vi "medicion.vi"(8 "Powermeter":T1={"Readout Config"="POW", "tiempo. lect."=0.0, "num. med"=0.0}, 9 "Config. fotodiodo":cluster{"tiempo. lect.":dbl, "num. med":dbl}, 10 "config. Polarizador":T2, 11 "Config. voltaje y corriente":T3 {"Measurement Function (0:Voltage)" items=["Voltage", "Current", "Power"]; "Unit(V)" items=["V", "mV", "kV", "A", "mA"]; "Function(0:Voltage)" items=["Voltage", "Current"]}) -> (0 "LockIn":dbl, 1 "Valor voltaje":dbl, 2 "Power meter":cluster{dbl[], dbl[]}(graph), 3 "Fototubo":cluster{dbl[], dbl[]}(graph), 4 "Readout value":dbl format="%^#_9e")   [LabVIEW 2016]
uses:
  <vilib>/Analysis/baseanly.llb/Mean (DBL).vi
  <instrlib>/Keithley 2200 Series/Keithley 2200 Series.lvlib
  <vilib>/Analysis/NI_AALBase.lvlib
panel:
  out "Readout string":string
  out "New":bool
  out "Error log":string
  in  "stop":bool
  out "name":string
  out "flags":bool[](array[boolean])
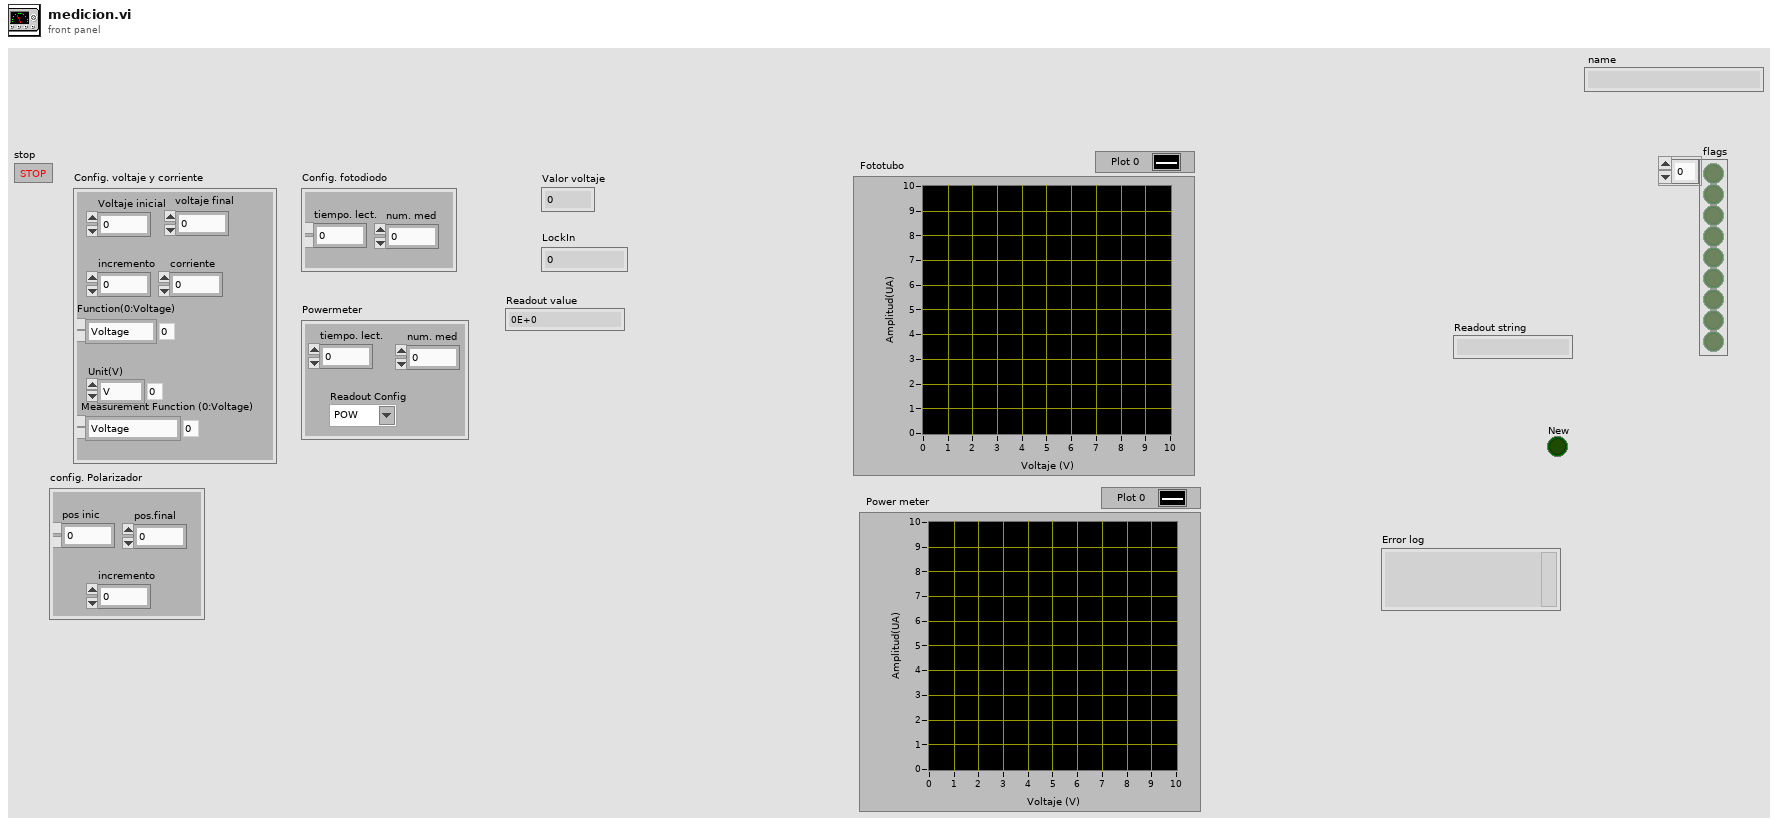
[diagram p1: front panel]
types:
  T1 = cluster{"Readout Config":string, "tiempo. lect.":dbl, "num. med":dbl}
  T2 = cluster{"pos inic":dbl, "pos.final":dbl, "incremento":dbl}
  T3 = cluster{"Voltaje inicial":dbl, "incremento":dbl, " voltaje final":dbl, "corriente":dbl, "Function(0:Voltage)":u16, "Unit(V)":u16, "Measurement Function (0:Voltage)":u16}
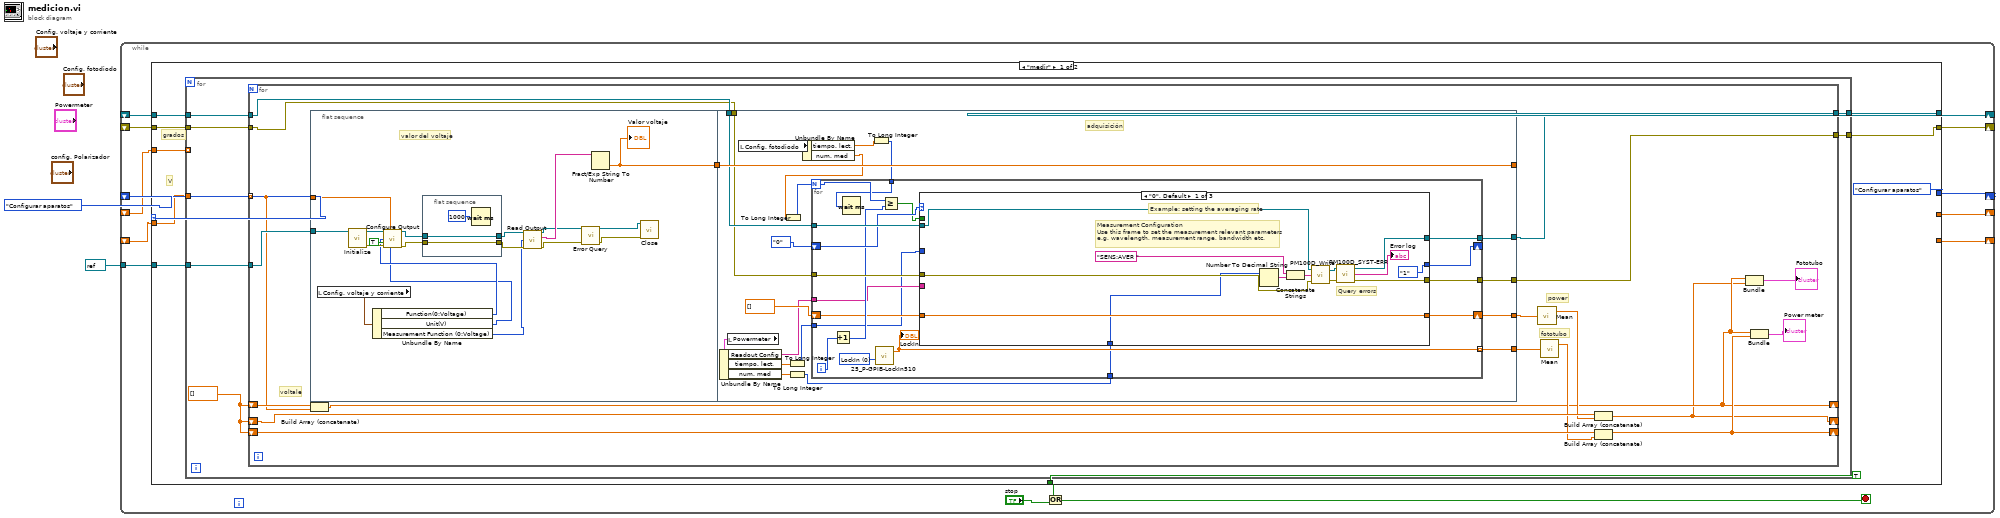
[diagram p0: block diagram]
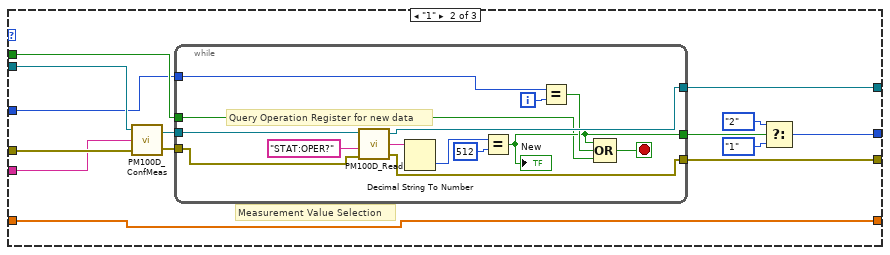
[diagram p2: hidden frame]
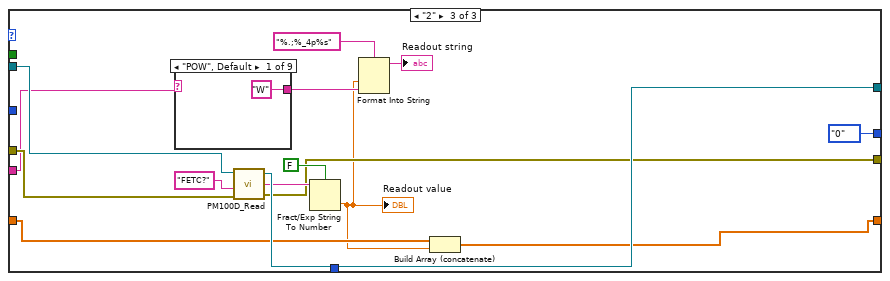
[diagram p3: hidden frame]
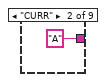
[diagram p4: hidden frame]
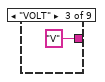
[diagram p5: hidden frame]
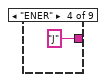
[diagram p6: hidden frame]
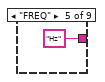
[diagram p7: hidden frame]
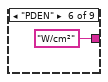
[diagram p8: hidden frame]
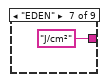
[diagram p9: hidden frame]
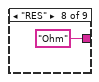
[diagram p10: hidden frame]
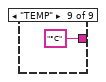
[diagram p11: hidden frame]
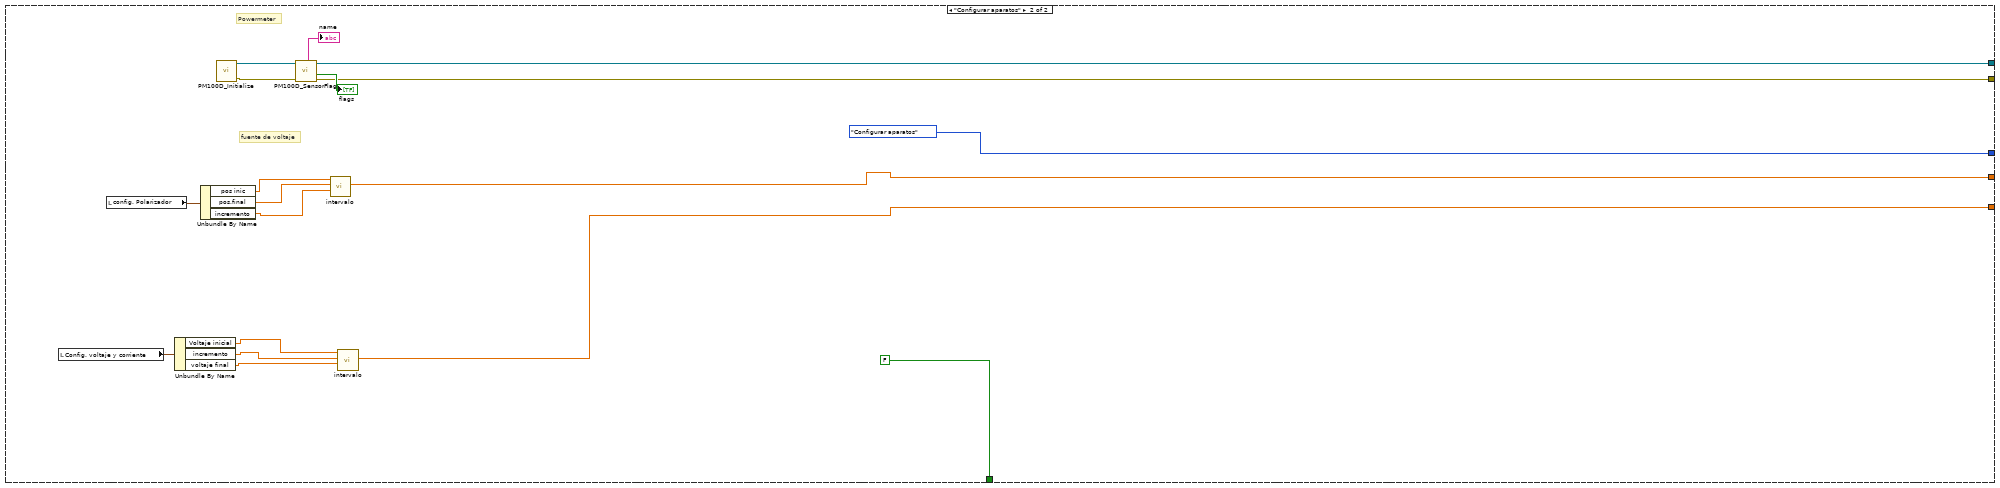
[diagram p12: hidden frame]
diagram:
  n1 = while {
    shift-right: [w3] -> _
    shift-left: enum16{"Configurar aparatos", "medir"}."Configurar aparatos" -> [w16]
    shift-right: [w15] -> _
    shift-left: _ -> [w9]
    shift-right: [w14] -> _
    shift-left: _ -> [w8]
    shift-right: [w13] -> _
    shift-left: _ -> [w11]
    shift-right: [w12] -> _
    shift-left: _ -> [w10]
    tunnel: refnum<visa-resource-name> refnum ("VISA resource name") -> [w4]
    stop <- w7 stop-if-true
    n2 = case shown="\"medir\"" w16 {
      tunnel: [w18 w184] -> w15
      tunnel: [w17 w183] -> w14
      tunnel: [_ w182] -> w13
      tunnel: [_ w181] -> w12
      tunnel: w11 -> [w25 _]
      tunnel: w10 -> [w24 _]
      tunnel: w9 -> [w23 _]
      tunnel: w8 -> [w22 _]
      tunnel: [TRUE FALSE] -> w5
      tunnel: w4 -> [w20 _]
      tunnel: [enum16{"Configurar aparatos", "medir"}."Configurar aparatos" enum16{"Configurar aparatos", "medir"}."Configurar aparatos"] -> w3
      frame "medir" {
        # "V"
        # "grados"
        n3 = for {
          tunnel: w25 -> [_] mode=indexing
          tunnel: w24 -> [w32]
          tunnel: w23 -> [w31]
          tunnel: w22 -> [w30]
          tunnel: w20 -> [w29]
          tunnel: [w27] -> w18
          tunnel: [w26] -> w17
          w28 = dbl[] []
          n4 = for {
            tunnel: w32 -> [w49] mode=indexing
            tunnel: w31 -> [w47]
            tunnel: w30 -> [w46]
            tunnel: w29 -> [w51]
            shift-right: [w34] -> _
            shift-left: w28 -> [w50]
            shift-right: [w33] -> _
            shift-left: w28 -> [w43]
            shift-right: [w36] -> _
            shift-left: w28 -> [w42]
            tunnel: [w39] -> w27
            tunnel: [w38] -> w26
            # "fototubo"
            # "power"
            # "voltale"
            n5 = flat-sequence {
              tunnel: w49 -> [w61]
              tunnel: w51 -> [w70]
              tunnel: [w60] -> w48
              tunnel: w48 -> [w93]
              tunnel: w47 -> [w89]
              tunnel: w46 -> [w88]
              tunnel: [w93] -> _
              tunnel: [w77] -> w45
              tunnel: [w76] -> w44
              tunnel: [w75] -> w39
              tunnel: [w74] -> w38
              frame #0 {
                # "valor del voltaje"
                n6 = local read "Config. voltaje y corriente"() -> (w59:T3)
                n7 = call <instrlib>:"Initialize.vi"("VISA resource name"=w70) -> ("error out"=w68:errorcluster, "VISA resource name out"=w69:refnum<visa-resource-name>)  [unwired: 9 in]
                n8 = Unbundle By Name(w59) -> ("Function(0:Voltage)"=w58:u16, "Unit(V)"=w57:u16, "Measurement Function (0:Voltage)"=w56:u16)
                n9 = call <instrlib>:"Configure Output.vi"("VISA resource name"=w69, "Manual Range(0.00)"=w61, "Function(0:Voltage)"=w58, "Enable Output (T: Enable)"=TRUE, "error in (no error)"=w68, "Unit(V)"=w57) -> ("VISA resource name out"=w66:refnum<visa-resource-name>, "error out"=w65:errorcluster)  [unwired: 8 in]
                n10 = flat-sequence {
                  tunnel: w65 -> [w72]
                  tunnel: [w72] -> w63
                  tunnel: w66 -> [w71]
                  tunnel: [w71] -> w64
                  frame #0 {
                    n11 = Wait (ms)(milliseconds to wait=u32 1000) -> ()  [unwired: 1 out]
                  }
                }
                n12 = call <instrlib>:"Read Output.vi"("VISA resource name"=w64, "Measurement Function (0:Voltage)"=w56, "error in (no error)"=w63) -> ("VISA resource name out"=w55:refnum<visa-resource-name>, "Measurement"=w62:string, "error out"=w54:errorcluster)  [unwired: 10 in]
                n13 = call <instrlib>:"Error Query.vi"("error in (no error)"=w54, "VISA resource name"=w55) -> ("error out"=w52:errorcluster, "VISA resource name out"=w53:refnum<visa-resource-name>)  [unwired: 6 in, 2 out]
                n14 = Fract/Exp String To Number(string=w62) -> (number=w60:dbl)  [unwired: 3 in, 1 out]
                "Valor voltaje" <- w60
                n15 = call <instrlib>:"Close.vi"("error in (no error)"=w52, "VISA resource name"=w53) -> ()  [unwired: 9 in, 1 out]
              }
              frame #1 {
                # "adquisición"
                n16 = local read "Powermeter"() -> (w85:T1)
                n17 = Unbundle By Name(w85) -> ("Readout Config"=w84:string, "tiempo. lect."=w83:dbl, "num. med"=w81:dbl)
                n18 = local read "Config. fotodiodo"() -> (w92:cluster{"tiempo. lect.":dbl, "num. med":dbl})
                n19 = To Long Integer(number=w81) -> (32bit integer=w80:i32)
                n20 = To Long Integer(number=w83) -> (32bit integer=w82:i32)
                n21 = Unbundle By Name(w92) -> ("tiempo. lect."=w91:dbl, "num. med"=w90:dbl)
                n22 = To Long Integer(number=w90) -> (32bit integer=w79:i32)
                n23 = To Long Integer(number=w91) -> (32bit integer=w78:i32)
                n24 = for {
                  N: w79 -> [w107]
                  shift-right: [w94] -> _
                  shift-left: enum16{"0", "1", "2"}."0" -> [w109]
                  tunnel: w89 -> [w111]
                  tunnel: w88 -> [w110]
                  shift-right: [w104] -> w77
                  shift-left: dbl[] [] -> [w103]
                  tunnel: [w101] -> w76 mode=indexing
                  tunnel: w84 -> [w100]
                  tunnel: w82 -> [w99]
                  tunnel: w80 -> [w98]
                  tunnel: w78 -> [w97]
                  tunnel: [w96] -> w75
                  tunnel: [w95] -> w74
                  i -> [w106]
                  w102 = u16 0 items=["LockIn", "LockIn-DMM"] ("Tipo")
                  n25 = Increment(x=w106) -> (x+1=w105:i32)
                  n26 = Wait (ms)(milliseconds to wait=w97) -> ()  [unwired: 1 out]
                  n27 = call "25_P-GPIB-LockIn510.vi"("Tipo"=w102) -> ("LockIn"=w101:dbl)  [unwired: 3 in, 1 out]
                  "LockIn" <- w101
                  n28 = Greater Or Equal?(x=w107, y=w105) -> (x >= y?=w108:bool)
                  n29 = case shown="\"0\", Default" w109 {
                    tunnel: w111 -> [w122 w138 w165]
                    tunnel: w110 -> [w117 w137 w164]
                    tunnel: [enum16{"0", "1", "2"}."1" w132 enum16{"0", "1", "2"}."0"] -> w94
                    tunnel: [w115 w134 w163] -> w96
                    tunnel: [w114 w133 w157] -> w95
                    tunnel: w108 -> [_ w128 _]
                    tunnel: w103 -> [w113 w127 w156]
                    tunnel: [w113 w127 w154] -> w104
                    tunnel: w100 -> [_ w126 w153]
                    tunnel: w99 -> [_ w125 _]
                    tunnel: w98 -> [w112 _ _]
                    frame "0", Default {
                      # "Query errors"
                      # "Example: setting the averaging rate"
                      # "Measurement Configuration\nUse this frame to set the measurement relevant parameters\ne.g. wavelength, measurement range, bandwidth etc."
                      n30 = Number To Decimal String(number=w112) -> (decimal integer string=w123:string)  [unwired: 1 in]
                      n31 = Concatenate Strings("SENS:AVER " ("string"), w123) -> (w121:string)
                      n32 = call "PM100D_Write.vi"("error in (no error)"=w117, "Command"=w121, "VISA in"=w122) -> ("error out"=w118:errorcluster, "VISA out"=w120:refnum<visa-resource-name>)
                      n33 = call "PM100D_SYST-ERR.vi"("error out 2"=w118, "VISA In"=w120) -> ("error out"=w114:errorcluster, "Error"=→"Error log":string, "VISA Out"=w115:refnum<visa-resource-name>)  [unwired: 1 in]
                    }
                    frame "1" {
                      # "Measurement Value Selection"
                      n34 = call "PM100D_ConfMeas.vi"("error in"=w137, "Conf:"=w126, "VISA In"=w138) -> ("error out"=w135:errorcluster, "dup VISA session"=w136:refnum<visa-resource-name>)
                      n35 = while {
                        tunnel: w136 -> [w148]
                        tunnel: w135 -> [w147]
                        tunnel: [w146] -> w134
                        tunnel: [w145] -> w133
                        tunnel: [w141] -> w129
                        tunnel: w128 -> [w140]
                        tunnel: w125 -> [w139]
                        i -> [w143]
                        stop <- w144 stop-if-true
                        # "Query Operation Register for new data"
                        n36 = call "PM100D_Read.vi"("error in (no error)"=w147, "Command"="STAT:OPER?", "VISA in"=w148) -> ("error out"=w145:errorcluster, "ReadValue"=w151:string, "VISA out"=w146:refnum<visa-resource-name>)  [unwired: 1 in]
                        n37 = Decimal String To Number(string=w151) -> (number=w150:i32)  [unwired: 2 in, 1 out]
                        n38 = Equal?(x=w150, y=512) -> (x = y?=w141:bool)
                        "New" <- w141
                        n39 = Equal?(x=w139, y=w143) -> (x = y?=w142:bool)
                        n40 = Compound Arithmetic op=OR(w141, w142, w140) -> (w144:bool)
                      }
                      n41 = Select(t=enum16{"0", "1", "2"}."2", s=w129, f=enum16{"0", "1", "2"}."1") -> (s? t:f=w132:enum16{"0", "1", "2"})
                    }
                    frame "2" {
                      n42 = case shown="\"POW\", Default" w153 {
                        tunnel: ["W" "A" "V" "J" "Hz" "W/cm²" "J/cm²" "Ohm" "°C"] -> w159
                        frame "POW", Default {
                        }
                        frame "CURR" {
                        }
                        frame "VOLT" {
                        }
                        frame "ENER" {
                        }
                        frame "FREQ" {
                        }
                        frame "PDEN" {
                        }
                        frame "EDEN" {
                        }
                        frame "RES" {
                        }
                        frame "TEMP" {
                        }
                      }
                      n43 = call "PM100D_Read.vi"("error in (no error)"=w164, "Command"="FETC?", "VISA in"=w165) -> ("error out"=w157:errorcluster, "ReadValue"=w162:string, "VISA out"=w163:refnum<visa-resource-name>)  [unwired: 1 in]
                      n44 = Fract/Exp String To Number(use system decimal point (T)=FALSE, string=w162) -> (number=w155:dbl)  [unwired: 2 in, 1 out]
                      "Readout value" <- w155
                      n45 = Format Into String(format string="%.;%_4p%s", w155, w159) -> (resulting string=→"Readout string":string)  [unwired: 2 in, 1 out]
                      n46 = Build Array (concatenate)(w156, w155) -> (w154:dbl[])
                    }
                  }
                }
              }
            }
            n47 = Build Array (concatenate)(w50, w49) -> (w34:dbl[])
            n48 = call-poly <vilib>:"Mean.vi"("X"=w45) -> ("mean"=w41:dbl)  [unwired: 1 out]
            n49 = call-poly <vilib>:"Mean.vi"("X"=w44) -> ("mean"=w40:dbl)  [unwired: 1 out]
            n50 = Build Array (concatenate)(w43, w41) -> (w33:dbl[])
            n51 = Build Array (concatenate)(w42, w40) -> (w36:dbl[])
            n52 = Bundle(w34, w33) -> (→"Fototubo":cluster{dbl[], dbl[]})  [unwired: 1 in]
            n53 = Bundle(w34, w36) -> (→"Power meter":cluster{dbl[], dbl[]})  [unwired: 1 in]
          }
        }
      }
      frame "Configurar aparatos" {
        # "fuente de voltaje"
        # "Powermeter"
        n54 = local read "Config. voltaje y corriente"() -> (w179:T3)
        n55 = local read "config. Polarizador"() -> (w180:T2)
        n56 = Unbundle By Name(w179) -> ("Voltaje inicial"=w187:dbl, "incremento"=w186:dbl, "voltaje final"=w185:dbl)
        n57 = Unbundle By Name(w180) -> ("pos inic"=w189:dbl, "pos.final"=w188:dbl, "incremento"=w190:dbl)
        n58 = call "PM100D_Initialize.vi"() -> ("error out"=w193:errorcluster, "VISA out"=w194:refnum<visa-resource-name>)  [unwired: 2 in, 2 out]
        n59 = call "PM100D_SensorFlag.vi"("error in (no error)"=w193, "VISA in"=w194) -> ("error out"=w183:errorcluster, "flags"=→"flags":bool[], "VISA out"=w184:refnum<visa-resource-name>, "name"=→"name":string)  [unwired: 2 in, 4 out]
        n60 = call "intervalo.vi"("incremento"=w190, "fin"=w188, "inicio"=w189) -> ("Array"=w182:dbl[])  [unwired: 8 in]
        n61 = call "intervalo.vi"("incremento"=w185, "fin"=w186, "inicio"=w187) -> ("Array"=w181:dbl[])  [unwired: 8 in]
      }
    }
    n62 = Or(x=w5, y="stop") -> (x .or. y?=w7:bool)
  }
